vi "Init_joe.vi"(0 "VISA resource":refnum<visa-resource-name>, 1 "Baud Rate (115200)":u32=115200, 2 "Board Type (Uno)":T3, 3 "Bytes Per Packet (15)":u32=15, 4 "Connection Type (USB/Serial)":T1, 5 "error in":errorcluster) -> (14 "Arduino Resource":T2={"VISA resource"="", "Board Type"=enum."Uno", "Connection Type"=enum."USB / Serial", "Bytes Per Packet (15)"=15}, 19 "error out":errorcluster)   [LabVIEW 2012]
doc: "Initializes a connection to an Arduino running the LabVIEW Interface for Arduino sketch.\n\nNote: The baud rate specified must match the baud rate defined by DEFAULTBAUDRATE in the Arduino firmware.\n\nNote: The Bytes Per Packet input must match the COMMANDLENGTH specified in the Arduino firmware."
uses:
  <vilib>/LabVIEW Interface for Arduino/Type Defs/Board Type.ctl
  <vilib>/LabVIEW Interface for Arduino/Type Defs/Arduino Resource.ctl
  <vilib>/LabVIEW Interface for Arduino/Type Defs/Connection Type.ctl
  <vilib>/Instr/_visa.llb/VISA Configure Serial Port (Instr).vi
  <vilib>/LabVIEW Interface for Arduino/LabVIEW Interface for Arduino.lvlib
panel:
  in  "MaxNumTimeouts (20)":u32=10
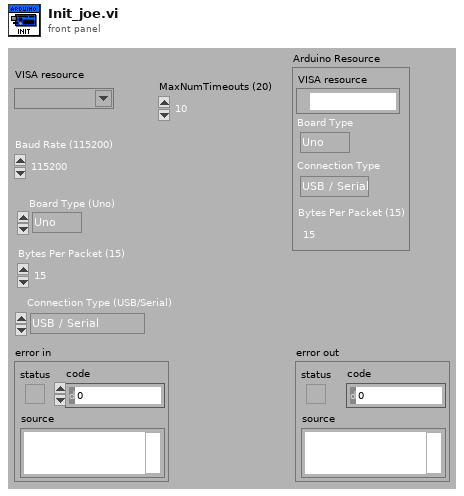
[diagram p1: front panel]
types:
  T1 = typedef "LabVIEW Interface for Arduino.lvlib/Connection Type.ctl" = enum8{"USB / Serial", "XBEE", "BlueSmirf (Bluetooth)"}
  T2 = typedef "LabVIEW Interface for Arduino.lvlib/Arduino Resource.ctl" = cluster{"VISA resource":refnum<visa-resource-name>, "Board Type":T3, "Connection Type":enum8{"USB / Serial"}, "Bytes Per Packet (15)":u8}
  T3 = typedef "LabVIEW Interface for Arduino.lvlib/Board Type.ctl" = enum16{"Uno", "Dimuelanove w/Atmega 328", "Mega 2560"}
  T4 = cluster{"VISA resource":refnum<visa-resource-name>, "Board Type (Uno)":T3, "Connection Type (USB/Serial)":T1, "Bytes Per Packet (15)":u32}
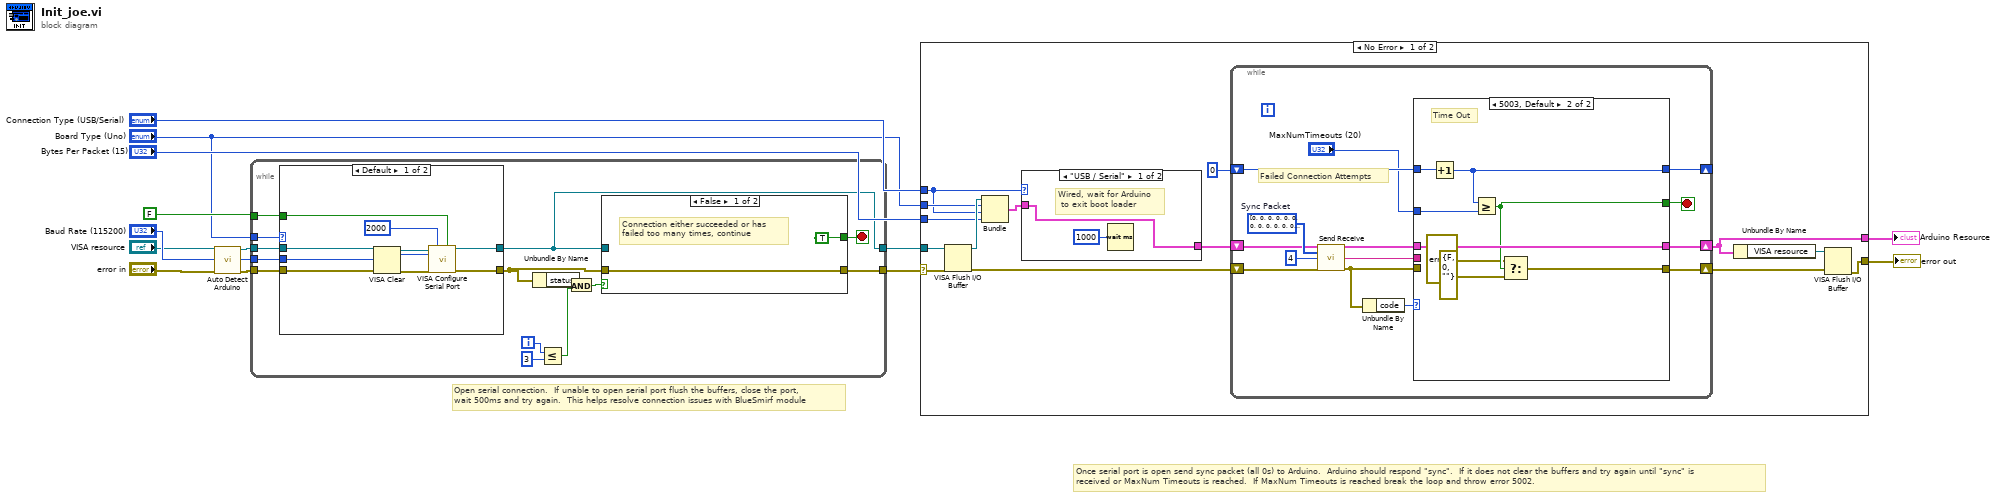
[diagram p0: block diagram]
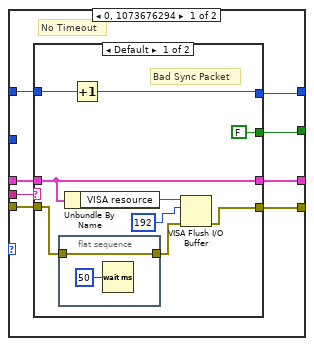
[diagram p3: hidden frame]
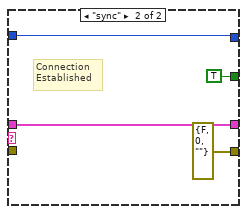
[diagram p4: hidden frame]
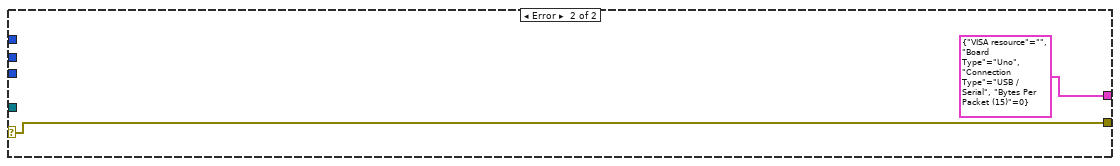
[diagram p5: hidden frame]
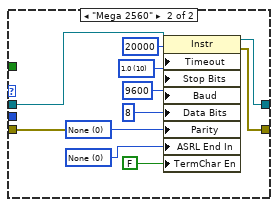
[diagram p6: hidden frame]
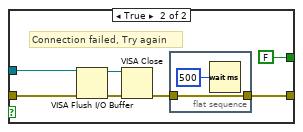
[diagram p7: hidden frame]
diagram:
  # "Once serial port is open send sync packet (all 0s) to Arduino.  Arduino should respond \"sync\".  If it does not clear the buffers and try again until \"sync\" is \nreceived or MaxNum Timeouts is reached.  If MaxNum Timeouts is reached break the loop and throw error 5002."
  # "Open serial connection.  If unable to open serial port flush the buffers, close the port,\nwait 500ms and try again.  This helps resolve connection issues with BlueSmirf module"
  n1 = call <vilib>:"Auto Detect Arduino.vi"("Visa Resource"="VISA resource", "error in (no error)"="error in") -> ("VISA resource"=w5:refnum<visa-resource-name>, "error out"=w3:errorcluster)  [unwired: 12 in]
  n2 = while {
    tunnel: FALSE ("Enable Termination\nChar (T)") -> [w27]
    tunnel: "Baud Rate (115200)" -> [w26]
    tunnel: w5 -> [w15]
    tunnel: [w19] -> w10
    tunnel: [w17] -> w9
    tunnel: w3 -> [w16]
    tunnel: "Board Type (Uno)" -> [w14]
    i -> [w24]
    stop <- w18 stop-if-true
    n3 = case shown="Default" w14 {
      tunnel: w27 -> [w36 _]
      tunnel: w26 -> [w35 _]
      tunnel: [w34 w37] -> w20
      tunnel: [w33 w38] -> w17
      tunnel: w16 -> [w31 w39]
      tunnel: w15 -> [w28 w40]
      frame Default {
        n4 = VISA Clear(VISA resource name=w28, error in (no error)=w31) -> (VISA resource name out=w29:refnum<visa-resource-name>, error out=w30:errorcluster)
        n5 = call-poly "VISA Configure Serial Port"("VISA resource name"=w29, "timeout (10sec)"=u32 2000, "Enable Termination\nChar (T)"=w36, "baud rate (9600)"=w35, "error in (no error)"=w30) -> ("VISA resource name out"=w33:refnum<visa-resource-name>, "error out"=w34:errorcluster)  [unwired: 9 in]
      }
      frame "Mega 2560" {
        w41 = u16 10 items=["1.0"=10, "1.5"=15, "2.0"=20] ("Serial Settings:Stop Bits")
        w44 = u16 0 items=["None", "Odd", "Even", "Mark", "Space"] ("Serial Settings:Parity")
        w45 = u16 0 items=["None", "Last Bit", "TermChar"] ("Serial Settings:End Mode for Reads")
        n6 = property class="Instr"(reference=w40, error in=w39, "Timeout"=u32 20000 ("General Settings:Timeout Value"), "Stop Bits"=w41, "Baud"=u32 9600 ("Serial Settings:Baud Rate"), "Data Bits"=u16 8 ("Serial Settings:Data Bits"), "Parity"=w44, "ASRL End In"=w45, "TermChar En"=FALSE ("Message Based Settings:Termination Character Enable")) -> (reference out=w38:refnum<visa-resource-name>, error out=w37:errorcluster)
      }
    }
    n7 = Unbundle By Name(w20) -> ("status"=w22:bool)
    n8 = Less Or Equal?(x=w24, y=3) -> (x <= y?=w23:bool)
    n9 = And(x=w22, y=w23) -> (x .and. y?=w21:bool)
    n10 = case shown="False" w21 {
      tunnel: w20 -> [w49 w52]
      tunnel: [w49 w51] -> w19
      tunnel: [TRUE FALSE] -> w18
      tunnel: w17 -> [_ w55]
      frame False {
        # "Connection either succeeded or has \nfailed too many times, continue"
      }
      frame True {
        # "Connection failed, Try again"
        n11 = VISA Flush I/O Buffer(VISA resource name=w55, error in (no error)=w52) -> (VISA resource name out=w54:refnum<visa-resource-name>, error out=w53:errorcluster)  [unwired: 1 in]
        n12 = VISA Close(VISA resource name=w54, error in (no error)=w53) -> (error out=w50:errorcluster)
        n13 = flat-sequence {
          tunnel: [w57] -> w51
          tunnel: w50 -> [w57]
          frame #0 {
            n14 = Wait (ms)(milliseconds to wait=u32 500) -> ()  [unwired: 1 out]
          }
        }
      }
    }
  }
  n15 = case shown="No Error" w10 {
    selector: w10 -> [w65 w122]
    tunnel: "Board Type (Uno)" -> [w62 _]
    tunnel: "Connection Type (USB/Serial)" -> [w61 _]
    tunnel: [w70 T2 {"VISA resource"="", "Board Type"=enum."Uno", "Connection Type"=enum."USB / Serial", "Bytes Per Packet (15)"=0} ("Arduino Resource")] -> w8
    tunnel: [w69 w122] -> w11
    tunnel: w9 -> [w67 _]
    tunnel: "Bytes Per Packet (15)" -> [w59 _]
    frame No Error {
      n16 = VISA Flush I/O Buffer(VISA resource name=w67, error in (no error)=w65) -> (VISA resource name out=w63:refnum<visa-resource-name>, error out=w68:errorcluster)  [unwired: 1 in]
      n17 = Bundle("VISA resource"=w63, "Board Type (Uno)"=w62, "Connection Type (USB/Serial)"=w61, "Bytes Per Packet (15)"=w59) -> (w60:T4)  [unwired: 1 in]
      n18 = case shown="\"USB / Serial\"" w61 {
        tunnel: w60 -> [w73 w75]
        tunnel: [w73 w75] -> w64
        frame "USB / Serial" {
          # "Wired, wait for Arduino\n to exit boot loader"
          n19 = Wait (ms)(milliseconds to wait=u32 1000) -> ()  [unwired: 1 out]
        }
        frame Default {
        }
      }
      n20 = while {
        shift-right: [w77] -> w70
        shift-left: w64 -> [w78]
        shift-right: [w82] -> w71
        shift-left: w68 -> [w89]
        shift-right: [w85] -> _
        shift-left: 0 -> [w84]
        stop <- w83 stop-if-true
        w88 = u8[] [0, 0, 0, 0, 0, 0, 0, 0, 0, 0, 0, 0, 0]  # Sync Packet
        # "Failed Connection Attempts"
        n21 = call <vilib>:"Send Receive.vi"("Arduino Resource"=w78, "Data"=w88, "Bytes To Read (0)"=u32 4, "error in"=w89) -> ("Arduino Resource"=w81:T2, "Read Buffer"=w80:string, "error out"=w79:errorcluster)  [unwired: 9 in]
        n22 = Unbundle By Name(w79) -> ("code"=w86:i32)
        n23 = case shown="5003, Default" w86 {
          tunnel: [w93 w119] -> w85
          tunnel: w84 -> [w92 w120]
          tunnel: [w90 w117] -> w83
          tunnel: [w96 w113] -> w82
          tunnel: [w95 w118] -> w77
          tunnel: w81 -> [w94 w118]
          tunnel: w80 -> [w97 _]
          tunnel: w79 -> [w91 _]
          tunnel: "MaxNumTimeouts (20)" -> [_ w116]
          frame 0, 1073676294 {
            # "No Timeout"
            n24 = case shown="Default" w97 {
              tunnel: [w101 errorcluster {"status"=FALSE, "code"=0, "source"=""} ("error out")] -> w96
              tunnel: [w103 w111] -> w95
              tunnel: w94 -> [w103 w111]
              tunnel: [FALSE TRUE] -> w90
              tunnel: w92 -> [w105 w109]
              tunnel: [w104 w109] -> w93
              tunnel: w91 -> [w100 _]
              frame Default {
                # "Bad Sync Packet"
                n25 = flat-sequence {
                  tunnel: w100 -> [w107]
                  tunnel: [w107] -> w99
                  frame #0 {
                    n26 = Wait (ms)(milliseconds to wait=u32 50) -> ()  [unwired: 1 out]
                  }
                }
                n27 = Unbundle By Name(w103) -> ("VISA resource"=w102:refnum<visa-resource-name>)
                n28 = Increment(x=w105) -> (x+1=w104:i32)
                n29 = VISA Flush I/O Buffer(VISA resource name=w102, mask (16)=u16 192, error in (no error)=w99) -> (error out=w101:errorcluster)  [unwired: 1 out]
              }
              frame "sync" {
                # "Connection \nEstablished"
              }
            }
          }
          frame 5003, Default {
            # "Time Out"
            n30 = Increment(x=w120) -> (x+1=w119:i32)
            n31 = Greater Or Equal?(x=w119, y=w116) -> (x >= y?=w117:bool)
            n32 = Select(t=errorcluster {"status"=TRUE, "code"=5002, "source"="Init.vi.  Unable to establish connection with Arduino.  Please ensure that you have selected the correct COM port and that you have flashed the Arduino with the correct firmware."} ("error out"), s=w117, f=errorcluster {"status"=FALSE, "code"=0, "source"=""}) -> (s? t:f=w113:errorcluster)
          }
        }
      }
      n33 = Unbundle By Name(w70) -> ("VISA resource"=w66:refnum<visa-resource-name>)
      n34 = VISA Flush I/O Buffer(VISA resource name=w66, error in (no error)=w71) -> (error out=w69:errorcluster)  [unwired: 1 in, 1 out]
    }
    frame Error {
    }
  }
  "error out" <- w11
  "Arduino Resource" <- w8
